vi "Channels Not Contiguous.vi"(8 "error in (no error)":errorcluster, 11 "name":string) -> (0 "error out":errorcluster)   [LabVIEW 2019, in "DSF Engine.lvlib" / "VeriStand DSF.lvclass"]
uses:
  VeriStand DSF.lvclass
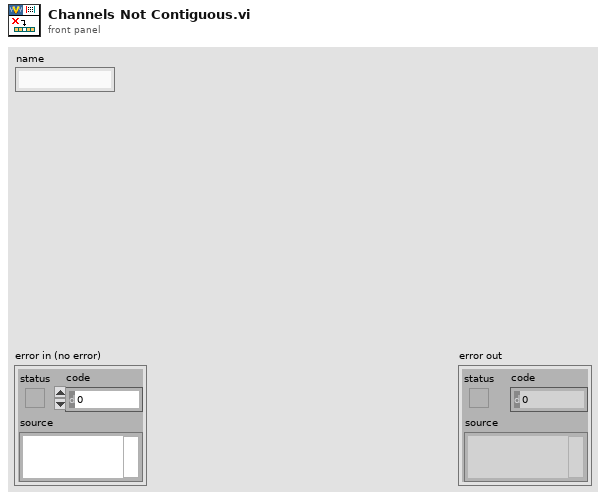
[diagram p1: front panel]
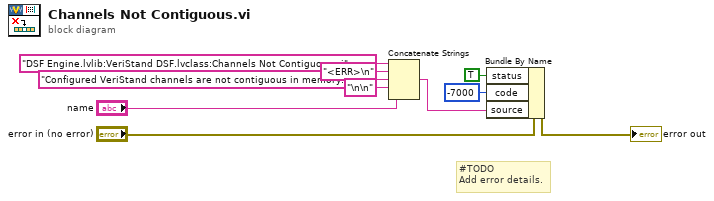
[diagram p0: block diagram]
diagram:
  # "#TODO\nAdd error details."
  n1 = Concatenate Strings("DSF Engine.lvlib:VeriStand DSF.lvclass:Channels Not Contiguous.vi" ("string"), "<ERR>\n", "Configured VeriStand channels are not contiguous in memory:" ("string"), "\n\n" ("string"), "name") -> (w3:string)
  n2 = Bundle By Name(cluster="error in (no error)", "status"=TRUE, "code"=-7000, "source"=w3) -> (→"error out":errorcluster)
